vi "test Set and Get Possible Endpoints.vi"(8 "error in (no error)":errorcluster, 11 "TestCase in":refnum<class "SLSC Switch Scripting Unit Tests.lvclass">) -> (0 "error out":errorcluster, 3 "TestCase out":refnum<class "SLSC Switch Scripting Unit Tests.lvclass">)   [LabVIEW 2017, in "SLSC Switch Scripting Unit Tests.lvclass"]
uses:
  SLSC Switch Scripting Unit Tests.lvclass
  <vilib>/addons/_JKI Toolkits/VI Tester/TestCase.llb/TestCase.lvclass
  NI-SWITCH Scripting.lvlib
  Custom Device/Find All SLSC Switch Custom Devices.vi
  Shared/Routing and Faulting Hardware API/Routing and Faulting Hardware API.lvlib
  Shared/Routing and Faulting Hardware API/Types/Possible Connections for Endpoint.ctl
  C:/Program Files (x86)/National Instruments/LabVIEW 2017/vi.lib/addons/_JKI Toolkits/VI Tester/TestCase.llb/TestCase.lvclass
panel:
  in  "Save?":bool
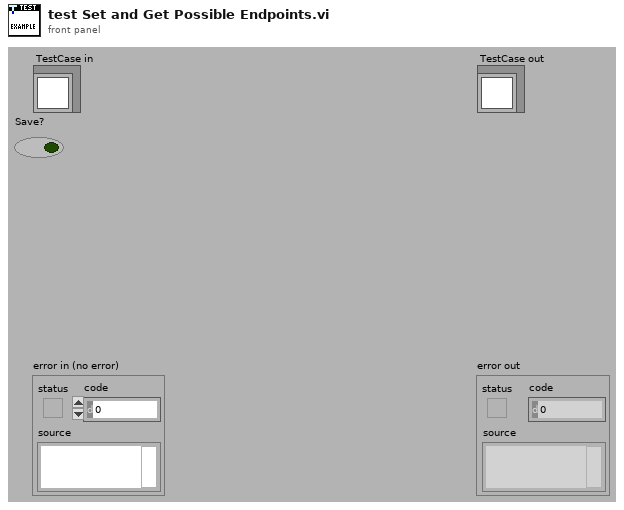
[diagram p1: front panel]
types:
  T1 = typedef "Routing and Faulting Hardware API.lvlib/Possible Connections for Endpoint.ctl" = cluster{"Source":string, "Destinations":string[]}
  T2 = typedef "Custom Device API.lvlib/Custom Device Item Ref.ctl" = u64
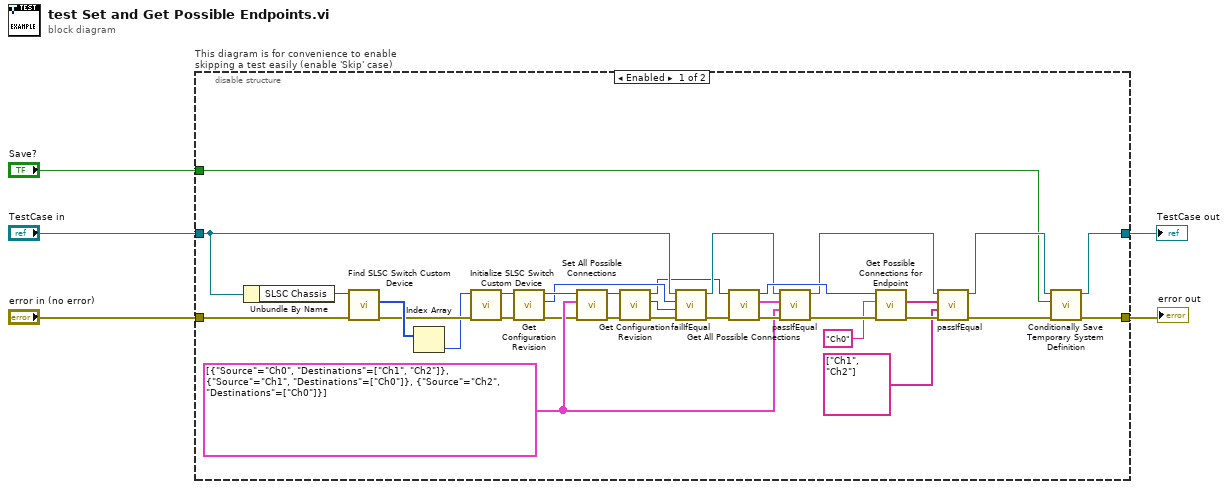
[diagram p0: block diagram]
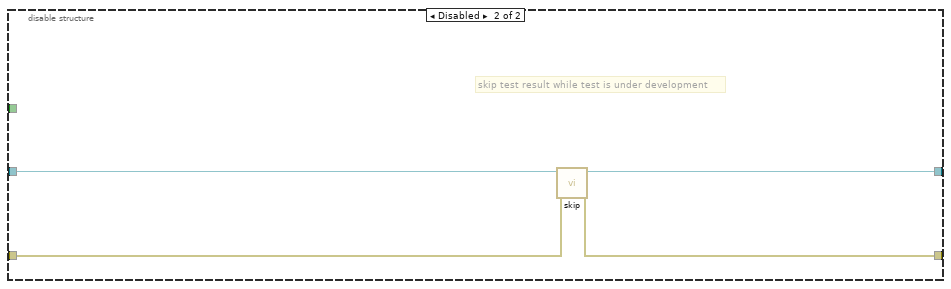
[diagram p2: hidden frame]
diagram:
  n1 = disable-structure "This diagram is for convenience to enable skipping a test easily (enable 'Skip' case)" shown="Enabled" {
    disable-tunnel: "TestCase in" -> [w11 w42]
    disable-tunnel: [w27 w40] -> w2
    disable-tunnel: [w26 w41] -> w4
    disable-tunnel: "error in (no error)" -> [w34 w39]
    disable-tunnel: "Save?" -> [w19 _]
    frame Enabled {
      w31 = T1[] [{"Source"="Ch0", "Destinations"=["Ch1", "Ch2"]}, {"Source"="Ch1", "Destinations"=["Ch0"]}, {"Source"="Ch2", "Destinations"=["Ch0"]}] ("Possible Connections")
      n2 = Unbundle By Name(w11) -> ("SLSC Chassis"=w35:u64)
      n3 = call-poly "Find SLSC Switch Custom Device.vi"("error in"=w34, "slsc chassis in"=w35) -> ("error out"=w37:errorcluster, "slsc switch custom devices"=w38:T2[])  [unwired: 7 in, 1 out]
      n4 = Index Array(array=w38) -> (element=w36:T2)  [unwired: 1 in]
      n5 = call "Initialize SLSC Switch Custom Device.vi"("error in"=w37, "slsc switch custom device in"=w36) -> ("error out"=w18:errorcluster, "slsc switch custom device out"=w17:T2)  [unwired: 7 in, 1 out]
      n6 = call "Get Configuration Revision.vi"("error in (no error)"=w18, "Hardware Ref in"=w17) -> ("error out"=w15:errorcluster, "Configuration Revision"=w7:u32, "Hardware Ref out"=w16:T2)  [unwired: 6 in, 1 out]
      n7 = call "Set All Possible Connections.vi"("error in (no error)"=w15, "Possible Connections"=w31, "Hardware Ref in"=w16) -> ("error out"=w14:errorcluster, "Hardware Ref out"=w13:T2)  [unwired: 7 in]
      n8 = call "Get Configuration Revision.vi"("error in (no error)"=w14, "Hardware Ref in"=w13) -> ("error out"=w12:errorcluster, "Configuration Revision"=w8:u32, "Hardware Ref out"=w6:T2)  [unwired: 6 in, 1 out]
      n9 = call-dynamic "failIfEqual.vi"("error in (no error)"=w12, "y"=w8, "x"=w7, "TestCase in"=w11) -> ("error out"=w9:errorcluster, "TestCase out"=w10:refnum<class "SLSC Switch Scripting Unit Tests.lvclass">)  [unwired: 6 in]
      n10 = call "Get All Possible Connections.vi"("error in (no error)"=w9, "Hardware Ref in"=w6) -> ("error out"=w33:errorcluster, "Possible Connections"=w32:T1[], "Hardware Ref out"=w29:T2)  [unwired: 6 in, 1 out]
      n11 = call-dynamic "passIfEqual.vi"("error in (no error)"=w33, "y"=w31, "x"=w32, "TestCase in"=w10) -> ("error out"=w30:errorcluster, "TestCase out"=w24:refnum<class "SLSC Switch Scripting Unit Tests.lvclass">)  [unwired: 6 in]
      n12 = call "Get Possible Connections for Endpoint.vi"("error in (no error)"=w30, "Endpoint"="Ch0", "Hardware Ref in"=w29) -> ("error out"=w22:errorcluster, "Possible Connections"=w25:string[])  [unwired: 6 in, 1 out]
      n13 = call-dynamic "passIfEqual.vi"("error in (no error)"=w22, "y"=string[] ["Ch1", "Ch2"] ("Destinations"), "x"=w25, "TestCase in"=w24) -> ("error out"=w21:errorcluster, "TestCase out"=w23:refnum<class "SLSC Switch Scripting Unit Tests.lvclass">)  [unwired: 6 in]
      n14 = call "Conditionally Save Temporary System Definition.vi"("error in (no error)"=w21, "Save?"=w19, "Test Case"=w23) -> ("error out"=w26:errorcluster, "Test Case"=w27:refnum<class "SLSC Switch Scripting Unit Tests.lvclass">)  [unwired: 6 in, 1 out]
    }
    frame Disabled {
      # "skip test result while test is under development"
      n15 = call <vilib>:"skip.vi"("error in (no error)"=w39, "TestCase in"=w42) -> ("error out"=w41:errorcluster, "TestCase out"=w40:refnum<class "SLSC Switch Scripting Unit Tests.lvclass">)  [unwired: 8 in]
    }
  }
  "error out" <- w4
  "TestCase out" <- w2
